vi "Charging_Wake-up Pulse.vi"(8 "error in (no error)":errorcluster, 9 "pulse width (ms)":u32=1000, 10 "pulses":i32=3) -> (0 "error out":errorcluster)   [LabVIEW 2010]
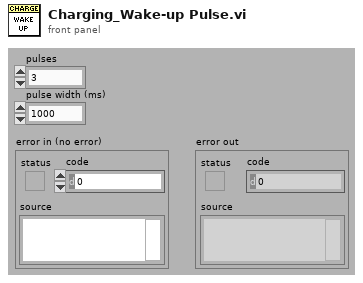
[diagram p1: front panel]
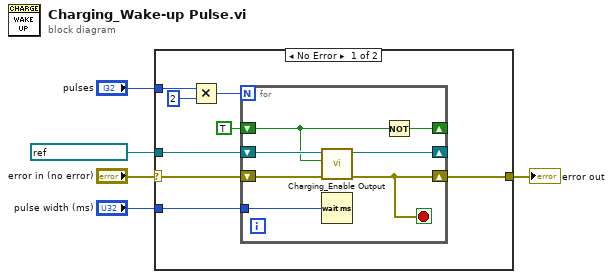
[diagram p0: block diagram]
diagram:
  n1 = case shown="No Error" "error in (no error)" {
    selector: "error in (no error)" -> [w7 w21]
    tunnel: refnum<k15> "IVI-AG33210A" ("instrument handle") -> [w8 _]
    tunnel: [w6 w21] -> w4
    tunnel: "pulse width (ms)" -> [w9 _]
    tunnel: "pulses" -> [w12 _]
    frame No Error {
      n2 = Multiply(x=w12, y=2) -> (x*y=w10:i32)
      n3 = for {
        N: w10 -> [_]
        shift-right: [w15] -> _
        shift-left: TRUE -> [w16]
        shift-right: [w18] -> w6
        shift-left: w7 -> [w20]
        tunnel: w9 -> [w17]
        shift-right: [w14] -> _
        shift-left: w8 -> [w19]
        stop <- w18 stop-if-true
        n4 = call "Charging_Enable Output.vi"("error in (no error)"=w20, "enable output (true)"=w16, "instrument handle"=w19) -> ("error out"=w18:errorcluster, "instrument handle out"=w14:refnum<k15>)  [unwired: 7 in]
        n5 = Wait (ms)(milliseconds to wait=w17) -> ()  [unwired: 1 out]
        n6 = Not(x=w16) -> (.not. x?=w15:bool)
      }
    }
    frame Error {
    }
  }
  "error out" <- w4
